vi "LaserSwitch.vi"(7 "error in (no error)":errorcluster, 9 "SwitchON?":bool=TRUE, 10 "reference In":refnum<k24>) -> (0 "error out":errorcluster, 3 "reference out":refnum<k24>)   [LabVIEW 2020]
doc: "Generates sample waveforms according to the signal type in the HW Config input."
uses:
  D:/Daguan/Development/RM21-MMicrosopeSource/HardwareAdapter/Lasers/Dependencies/Oxxius_Boxx.dll
  Dependencies/Oxxius_Boxx.dll
  Global.vi
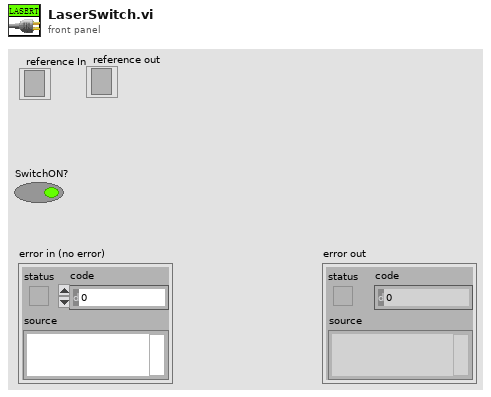
[diagram p1: front panel]
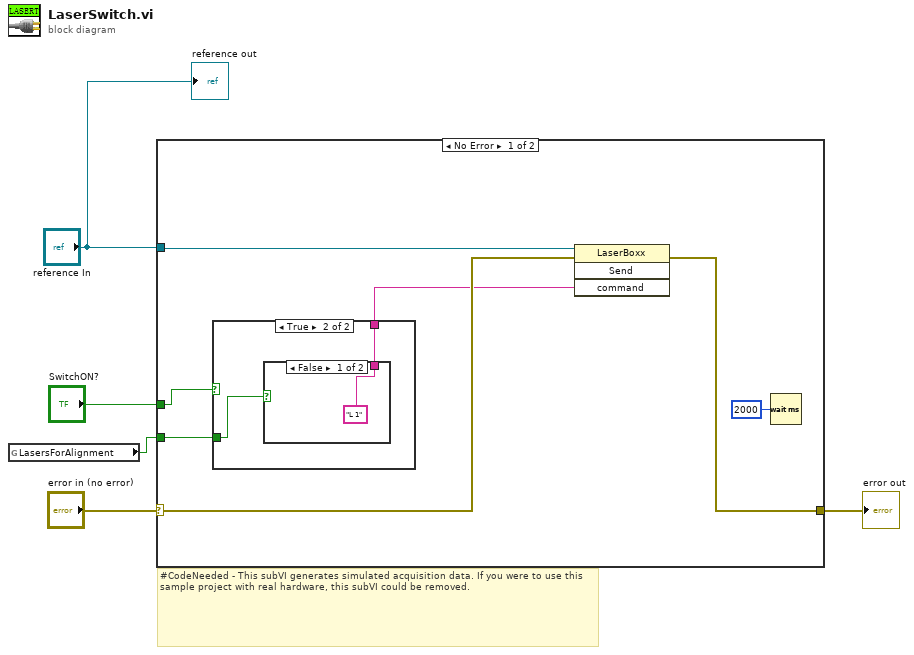
[diagram p0: block diagram]
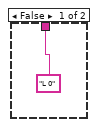
[diagram p2: hidden frame]
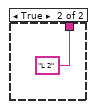
[diagram p3: hidden frame]
diagram:
  # "#CodeNeeded - This subVI generates simulated acquisition data. If you were to use this sample project with real hardware, this subVI could be removed."
  n1 = global read "Global.vi" "LasersForAlignment"() -> (w1:bool)
  n2 = case shown="No Error" "error in (no error)" {
    selector: "error in (no error)" -> [w11 w18]
    tunnel: [w12 w18] -> w4
    tunnel: "reference In" -> [w9 _]
    tunnel: "SwitchON?" -> [w8 _]
    tunnel: w1 -> [w7 _]
    frame No Error {
      n3 = case shown="True" w8 {
        tunnel: ["L 0" ("command") w15] -> w10
        tunnel: w7 -> [_ w14]
        frame False {
        }
        frame True {
          n4 = case shown="False" w14 {
            tunnel: ["L 1" ("command") "L 2" ("command")] -> w15
            frame False {
            }
            frame True {
            }
          }
        }
      }
      n5 = invoke class="LaserBoxx" method="Send"(reference=w9, error in=w11, "command"=w10) -> (error out=w12:errorcluster)  [unwired: 1 in, 3 out]
      n6 = Wait (ms)(milliseconds to wait=u32 2000) -> ()  [unwired: 1 out]
    }
    frame Error {
    }
  }
  "error out" <- w4
  "reference out" <- "reference In"
